vi "Event Keygen.vi"(8 "error in (no error)":errorcluster, 11 "[MV] Key Generator in":refnum<class "[MV] Key Generator.lvclass">) -> (0 "error out":errorcluster, 3 "[MV] Key Generator out":refnum<class "[MV] Key Generator.lvclass">)   [LabVIEW 2020, in "[MV] Key Generator.lvlib" / "[MV] Key Generator.lvclass"]
uses:
  [MV] Key Generator.lvclass
  <vilib>/regexp/Match Regular Expression.xnode
  <vilib>/YU/YU_Encrypt/AES/AES.lvclass
  <vilib>/YU/YU_Encrypt/RSA/RSA.lvclass
  <vilib>/YU/YU_Encrypt/Base64/Base64.lvclass
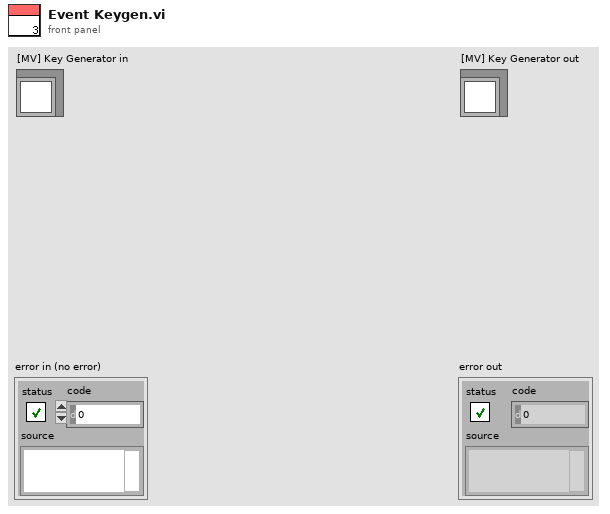
[diagram p1: front panel]
types:
  T1 = cluster{"machine_code":string, "sign_time":u64, "valid_days":i16}
  T2 = map{string, cluster{"private":string, "public":string}}
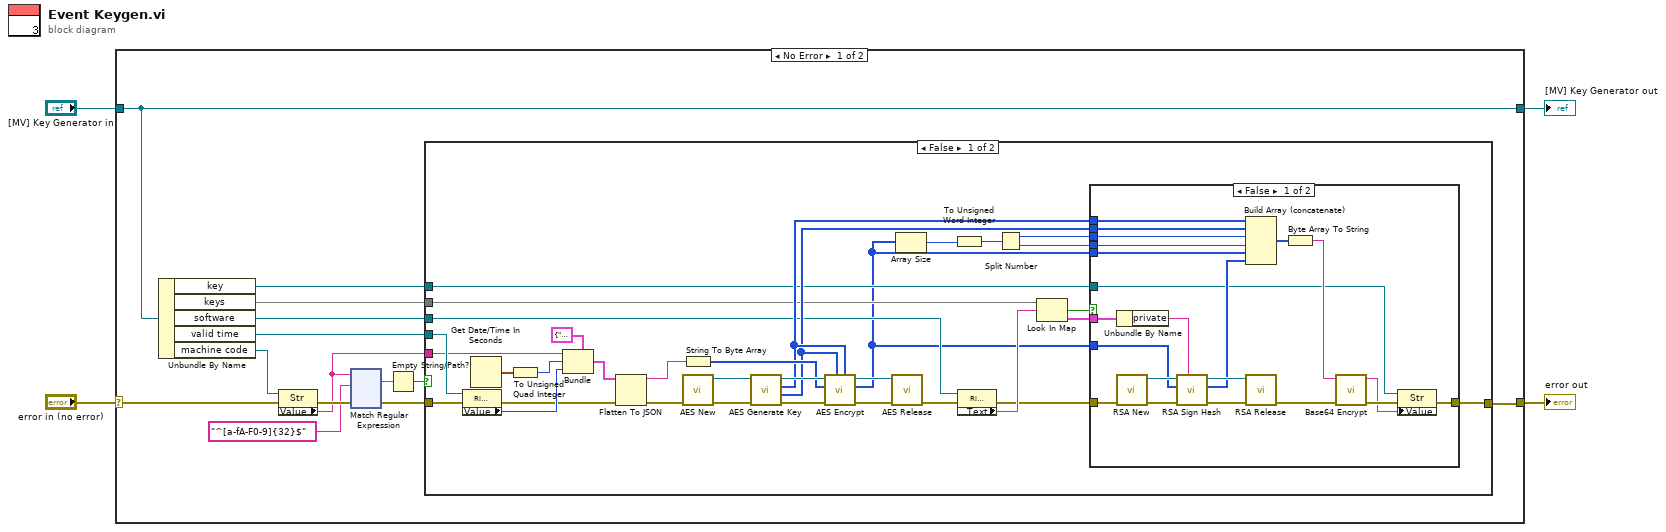
[diagram p0: block diagram]
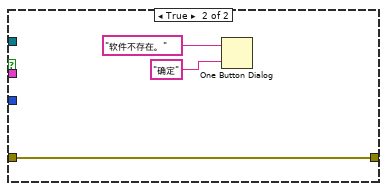
[diagram p2: hidden frame]
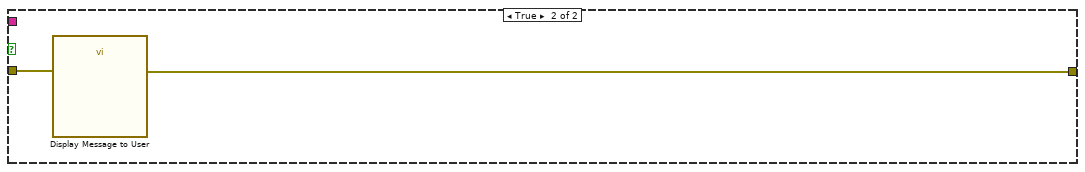
[diagram p3: hidden frame]
diagram:
  n1 = case shown="No Error" "error in (no error)" {
    selector: "error in (no error)" -> [w17 w197]
    tunnel: [w10 w197] -> w3
    tunnel: [w18 w196] -> w1
    tunnel: "[MV] Key Generator in" -> [w18 w196]
    frame No Error {
      n2 = Unbundle By Name(w18) -> ("key"=w5:refnum<vi>, "keys"=w6:T2, "software"=w7:refnum<vi>, "valid time"=w8:refnum<vi>, "machine code"=w16:refnum<vi>)
      n3 = property class="Str"(reference=w16, error in=w17) -> (error out=w15:errorcluster, "Value"=w9:string)  [unwired: 1 out]
      n4 = xnode "Match Regular Expression"("input string"=w9, "regular expression"="^[a-fA-F0-9]{32}$", "error in"=w15) -> ("whole match"=w13:string, "error out"=w11:errorcluster)  [unwired: 3 in, 3 out]
      n5 = Empty String/Path?(string/path=w13) -> (empty?=w12:bool)
      n6 = case shown="False" w12 {
        tunnel: w11 -> [w52 w78]
        tunnel: [w21 w77] -> w10
        tunnel: w9 -> [w49 _]
        tunnel: w8 -> [w51 _]
        tunnel: w7 -> [w27 _]
        tunnel: w6 -> [w26 _]
        tunnel: w5 -> [w22 _]
        frame False {
          n7 = property class="Ring (strict)"(reference=w51, error in=w52) -> (error out=w45:errorcluster, "Value"=w46:i16)  [unwired: 1 out]
          n8 = Get Date/Time In Seconds() -> (seconds since 1Jan1904=w48:timestamp)
          n9 = To Unsigned Quad Integer(1:w48) -> (0:w47:u64)
          n10 = Bundle(cluster=T1 {"machine_code"="", "sign_time"=0, "valid_days"=0}, "machine_code"=w49, "sign_time"=w47, "valid_days"=w46) -> (w44:T1)
          n11 = Flatten To JSON(anything=w44, error in (no error)=w45) -> (JSON string=w38:string, 11:w43:errorcluster)  [unwired: 1 in]
          n12 = String To Byte Array(string=w38) -> (unsigned byte array=w37:u8[])
          n13 = call <vilib>:"AES New.vi"("error in (no error)"=w43) -> ("error out"=w42:errorcluster, "AES out"=w41:refnum<class "AES.lvclass">)  [unwired: 9 in]
          n14 = call <vilib>:"AES Generate Key.vi"("error in (no error)"=w42, "AES in"=w41) -> ("error out"=w40:errorcluster, "IV"=w33:u8[], "Key"=w34:u8[], "AES out"=w39:refnum<class "AES.lvclass">)  [unwired: 6 in]
          n15 = call <vilib>:"AES Encrypt.vi"("Key"=w34, "IV"=w33, "error in (no error)"=w40, "data"=w37, "AES in"=w39) -> ("error out"=w36:errorcluster, "encrypted_data"=w19:u8[], "AES out"=w35:refnum<class "AES.lvclass">)  [unwired: 4 in]
          n16 = call <vilib>:"AES Release.vi"("error in (no error)"=w36, "AES in"=w35) -> ("error out"=w28:errorcluster)  [unwired: 9 in]
          n17 = Array Size(array=w19) -> (size(s)=w32:i32)
          n18 = To Unsigned Word Integer(number=w32) -> (unsigned 16bit integer=w31:u16)
          n19 = property class="Ring (strict)"(reference=w27, error in=w28) -> (error out=w24:errorcluster, "RingText.Text"=w25:string)  [unwired: 1 out]
          n20 = Split Number(x=w31) -> (hi(x)=w30:u8, lo(x)=w29:u8)
          n21 = Look In Map(map=w26, key=w25) -> (key not found?=w20:bool, value=w23:cluster{"private":string, "public":string})  [unwired: 1 in]
          n22 = case shown="False" w20 {
            tunnel: w34 -> [w73 _]
            tunnel: w33 -> [w72 _]
            tunnel: w30 -> [w71 _]
            tunnel: w29 -> [w70 _]
            tunnel: w19 -> [w67 _]
            tunnel: w24 -> [w64 w76]
            tunnel: w23 -> [w63 _]
            tunnel: w22 -> [w56 _]
            tunnel: [w54 w76] -> w21
            tunnel: w19 -> [w53 _]
            frame False {
              n23 = Unbundle By Name(w63) -> ("private"=w62:string)
              n24 = call <vilib>:"RSA New.vi"("error in (no error)"=w64) -> ("error out"=w69:errorcluster, "RSA out"=w68:refnum<class "RSA.lvclass">)  [unwired: 9 in]
              n25 = call <vilib>:"RSA Sign Hash.vi"("private_key"=w62, "error in (no error)"=w69, "data"=w53, "RSA in"=w68) -> ("error out"=w66:errorcluster, "signed_data"=w61:u8[], "RSA out"=w65:refnum<class "RSA.lvclass">)  [unwired: 5 in]
              n26 = Build Array (concatenate)(w73, w72, w71, w70, w67, w61) -> (w59:u8[])
              n27 = call <vilib>:"RSA Release.vi"("error in (no error)"=w66, "RSA in"=w65) -> ("error out"=w60:errorcluster)  [unwired: 9 in]
              n28 = Byte Array To String(unsigned byte array=w59) -> (string=w58:string)
              n29 = call <vilib>:"Base64 Encrypt.vi"("error in (no error)"=w60, "message"=w58) -> ("error out"=w57:errorcluster, "message_encrypted"=w55:string)  [unwired: 8 in]
              n30 = property class="Str"(reference=w56, error in=w57, "Value"=w55) -> (error out=w54:errorcluster)  [unwired: 1 out]
            }
            frame True {
              n31 = One Button Dialog(message="软件不存在。", button name ("OK")="确定") -> ()  [unwired: 1 out]
            }
          }
        }
        frame True {
          n32 = call "Display Message to User"("error in (no error)"=w78) -> ("error out"=w77:errorcluster)  [unwired: 9 in, 1 out]
        }
      }
    }
    frame Error {
    }
  }
  "error out" <- w3
  "[MV] Key Generator out" <- w1
